vi "9045_sm.vi"() -> ()   [LabVIEW 2020]
uses:
  controls/sm_cluster.ctl
  controls/enum.ctl
  lib/labviewRT-EPICS/sm bool read and increment.vi
  lib/labviewRT-EPICS/sm bool write and increment.vi
  lib/labviewRT-EPICS/sm bool array write and increment.vi
  lib/labviewRT-EPICS/sm double read and increment.vi
  lib/labviewRT-EPICS/sm double write and increment.vi
  lib/labviewRT-EPICS/sm double array write and increment.vi
  lib/labviewRT-EPICS/sm i8 read and increment.vi
  lib/labviewRT-EPICS/sm i8 write and increment.vi
  lib/labviewRT-EPICS/sm i8 write array and increment.vi
  lib/labviewRT-EPICS/sm i16 read and increment.vi
  lib/labviewRT-EPICS/sm i16 write and increment.vi
  lib/labviewRT-EPICS/sm i16 write array and increment.vi
  lib/labviewRT-EPICS/sm i32 read and increment.vi
  lib/labviewRT-EPICS/sm i32 write and increment.vi
  lib/labviewRT-EPICS/sm i32 write array and increment.vi
  lib/labviewRT-EPICS/sm i64 read and increment.vi
  lib/labviewRT-EPICS/sm i64 write and increment.vi
  lib/labviewRT-EPICS/sm i64 write array and increment.vi
  lib/labviewRT-EPICS/sm single read and increment.vi
  lib/labviewRT-EPICS/sm single write and increment.vi
  lib/labviewRT-EPICS/sm single array write and increment.vi
  lib/labviewRT-EPICS/sm u8 read and increment.vi
  lib/labviewRT-EPICS/sm u8 write and increment.vi
  lib/labviewRT-EPICS/sm u8 write array and increment.vi
  lib/labviewRT-EPICS/sm u16 read and increment.vi
  lib/labviewRT-EPICS/sm u16 write and increment.vi
  lib/labviewRT-EPICS/sm u16 write array and increment.vi
  lib/labviewRT-EPICS/sm u32 read and increment.vi
  lib/labviewRT-EPICS/sm u32 write and increment.vi
  lib/labviewRT-EPICS/sm u32 write array and increment.vi
  lib/labviewRT-EPICS/sm u64 read and increment.vi
  lib/labviewRT-EPICS/sm u64 write and increment.vi
  lib/labviewRT-EPICS/sm u64 write array and increment.vi
  lib/labviewRT-EPICS/sm mbbi write and increment.vi
  lib/labviewRT-EPICS/sm mbbo read and increment.vi
  lib/labviewRT-EPICS/linuxSharedMemory.lvlib
panel:
  in  "d40":T1
  out "d41":T1
  out "d37":u64
  in  "d38":u64
  in  "d39":u64[](array[numeric])
  out "d34":u32
  in  "d35":u32
  in  "d36":u32[](array[numeric])
  out "d30":u16
  in  "d31":u16
  in  "d32":u16[](array[numeric])
  out "d26":u8
  in  "d27":u8
  in  "d28":u8[](array[numeric])
  out "d22":sgl format="%.2f"
  in  "d23":sgl
  in  "d24":sgl[](array[numeric])
  out "d18":i64
  in  "d19":i64
  in  "d20":i64[](array[numeric])
  out "d14":i32
  in  "d15":i32
  in  "d16":i32[](array[numeric])
  out "d10":i16
  in  "d11":i16
  in  "d12":i16[](array[numeric])
  out "d6":i8
  in  "d7":i8
  in  "d8":i8[](array[numeric])
  in  "d4":dbl[](array[numeric])
  in  "d3":dbl
  out "d2":dbl
  in  "boolArrayWrite":bool[](array[boolean])
  in  "value in":bool
  out "Shared memory cluster":T2
  out "Bool out":bool
  in  "stop":bool
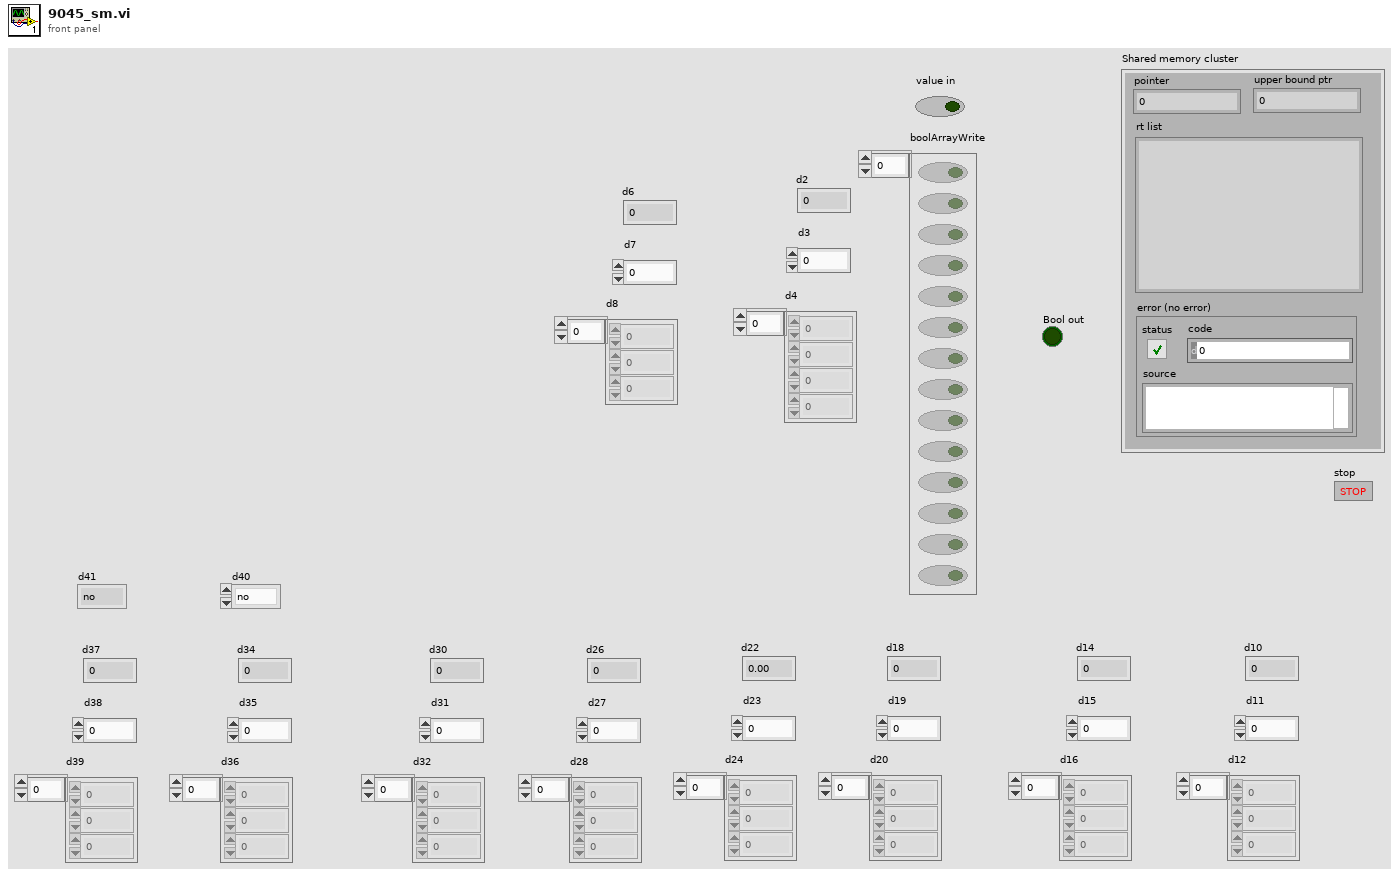
[diagram p1: front panel]
types:
  T1 = typedef "enum.ctl" = enum16{"no", "yes", "dont know"}
  T2 = typedef "linuxSharedMemory.lvlib/sm_cluster.ctl" = cluster{"rt list":string, "error (no error)":errorcluster, "pointer":u64, "upper bound ptr":u64}
  T3 = typedef "Linux RT IPC.Shared Memory.lvlib/reference.ctl" = refnum<data-value>
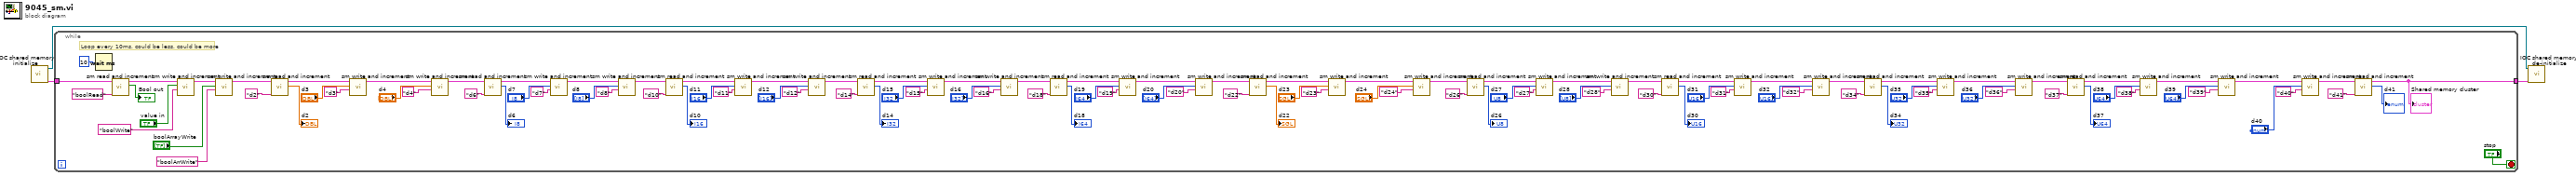
[diagram p0: block diagram]
diagram:
  n1 = call "IOC shared memory initialize.vi"() -> ("Shared memory cluster"=w2:T2, "shared memory class"=w3:T3)  [unwired: 10 in]
  n2 = while {
    tunnel: w2 -> [w21]
    tunnel: [w6] -> w1
    stop <- "stop" stop-if-true
    # "Loop every 10ms, could be less, could be more"
    n3 = Wait (ms)(milliseconds to wait=10) -> ()  [unwired: 1 out]
    n4 = call-poly "sm read and increment.vi"("Identifier"="boolRead", "Shared memory cluster input"=w21) -> ("Bool out"=→"Bool out":bool, "Shared memory cluster output"=w107:T2)  [unwired: 8 in]
    n5 = call-poly "sm write and increment.vi"("Identifier"="boolWrite", "value in"="value in", "Shared memory cluster input"=w107) -> ("Shared memory cluster output"=w104:T2)  [unwired: 8 in]
    n6 = call-poly "sm write and increment.vi"("Identifier"="boolArrWrite", "value in"="boolArrayWrite", "Shared memory cluster"=w104) -> ("Shared memory cluster output"=w20:T2)  [unwired: 8 in]
    n7 = call-poly "sm read and increment.vi"("Identifier"="d2", "Shared memory cluster input"=w20) -> ("Value out"=→"d2":dbl, "Shared memory cluster output"=w100:T2)  [unwired: 8 in]
    n8 = call-poly "sm write and increment.vi"("Identifier"="d3", "value in"="d3", "Shared memory cluster input"=w100) -> ("Shared memory cluster output"=w101:T2)  [unwired: 8 in]
    n9 = call-poly "sm write and increment.vi"("Identifier"="d4", "value in"="d4", "Shared memory cluster"=w101) -> ("Shared memory cluster output"=w19:T2)  [unwired: 8 in]
    n10 = call-poly "sm read and increment.vi"("Identifier"="d6", "Shared memory cluster input"=w19) -> ("Value out"=→"d6":i8, "Shared memory cluster output"=w92:T2)  [unwired: 8 in]
    n11 = call-poly "sm write and increment.vi"("Identifier"="d7", "value in"="d7", "Shared memory cluster input"=w92) -> ("Shared memory cluster output"=w93:T2)  [unwired: 8 in]
    n12 = call-poly "sm write and increment.vi"("Identifier"="d8", "value in"="d8", "Shared memory cluster"=w93) -> ("Shared memory cluster output"=w18:T2)  [unwired: 8 in]
    n13 = call-poly "sm read and increment.vi"("Identifier"="d10", "Shared memory cluster input"=w18) -> ("Value out"=→"d10":i16, "Shared memory cluster output"=w84:T2)  [unwired: 8 in]
    n14 = call-poly "sm write and increment.vi"("Identifier"="d11", "value in"="d11", "Shared memory cluster input"=w84) -> ("Shared memory cluster output"=w85:T2)  [unwired: 8 in]
    n15 = call-poly "sm write and increment.vi"("Identifier"="d12", "value in"="d12", "Shared memory cluster"=w85) -> ("Shared memory cluster output"=w17:T2)  [unwired: 8 in]
    n16 = call-poly "sm read and increment.vi"("Identifier"="d14", "Shared memory cluster input"=w17) -> ("Value out"=→"d14":i32, "Shared memory cluster output"=w76:T2)  [unwired: 8 in]
    n17 = call-poly "sm write and increment.vi"("Identifier"="d15", "value in"="d15", "Shared memory cluster input"=w76) -> ("Shared memory cluster output"=w77:T2)  [unwired: 8 in]
    n18 = call-poly "sm write and increment.vi"("Identifier"="d16", "value in"="d16", "Shared memory cluster"=w77) -> ("Shared memory cluster output"=w16:T2)  [unwired: 8 in]
    n19 = call-poly "sm read and increment.vi"("Identifier"="d18", "Shared memory cluster input"=w16) -> ("Value out"=→"d18":i64, "Shared memory cluster output"=w68:T2)  [unwired: 8 in]
    n20 = call-poly "sm write and increment.vi"("Identifier"="d19", "value in"="d19", "Shared memory cluster input"=w68) -> ("Shared memory cluster output"=w69:T2)  [unwired: 8 in]
    n21 = call-poly "sm write and increment.vi"("Identifier"="d20", "value in"="d20", "Shared memory cluster"=w69) -> ("Shared memory cluster output"=w15:T2)  [unwired: 8 in]
    n22 = call-poly "sm read and increment.vi"("Identifier"="d22", "Shared memory cluster input"=w15) -> ("Value out"=→"d22":sgl, "Shared memory cluster output"=w60:T2)  [unwired: 8 in]
    n23 = call-poly "sm write and increment.vi"("Identifier"="d23", "value in"="d23", "Shared memory cluster input"=w60) -> ("Shared memory cluster output"=w61:T2)  [unwired: 8 in]
    n24 = call-poly "sm write and increment.vi"("Identifier"="d24", "value in"="d24", "Shared memory cluster"=w61) -> ("Shared memory cluster output"=w14:T2)  [unwired: 8 in]
    n25 = call-poly "sm read and increment.vi"("Identifier"="d26", "Shared memory cluster input"=w14) -> ("Value out"=→"d26":u8, "Shared memory cluster output"=w52:T2)  [unwired: 8 in]
    n26 = call-poly "sm write and increment.vi"("Identifier"="d27", "value in"="d27", "Shared memory cluster input"=w52) -> ("Shared memory cluster output"=w53:T2)  [unwired: 8 in]
    n27 = call-poly "sm write and increment.vi"("Identifier"="d28", "value in"="d28", "Shared memory cluster"=w53) -> ("Shared memory cluster output"=w13:T2)  [unwired: 8 in]
    n28 = call-poly "sm read and increment.vi"("Identifier"="d30", "Shared memory cluster input"=w13) -> ("Value out"=→"d30":u16, "Shared memory cluster output"=w44:T2)  [unwired: 8 in]
    n29 = call-poly "sm write and increment.vi"("Identifier"="d31", "value in"="d31", "Shared memory cluster input"=w44) -> ("Shared memory cluster output"=w45:T2)  [unwired: 8 in]
    n30 = call-poly "sm write and increment.vi"("Identifier"="d32", "value in"="d32", "Shared memory cluster"=w45) -> ("Shared memory cluster output"=w11:T2)  [unwired: 8 in]
    n31 = call-poly "sm read and increment.vi"("Identifier"="d34", "Shared memory cluster input"=w11) -> ("Value out"=→"d34":u32, "Shared memory cluster output"=w36:T2)  [unwired: 8 in]
    n32 = call-poly "sm write and increment.vi"("Identifier"="d35", "value in"="d35", "Shared memory cluster input"=w36) -> ("Shared memory cluster output"=w37:T2)  [unwired: 8 in]
    n33 = call-poly "sm write and increment.vi"("Identifier"="d36", "value in"="d36", "Shared memory cluster"=w37) -> ("Shared memory cluster output"=w12:T2)  [unwired: 8 in]
    n34 = call-poly "sm read and increment.vi"("Identifier"="d37", "Shared memory cluster input"=w12) -> ("Value out"=→"d37":u64, "Shared memory cluster output"=w28:T2)  [unwired: 8 in]
    n35 = call-poly "sm write and increment.vi"("Identifier"="d38", "value in"="d38", "Shared memory cluster input"=w28) -> ("Shared memory cluster output"=w29:T2)  [unwired: 8 in]
    n36 = call-poly "sm write and increment.vi"("Identifier"="d39", "value in"="d39", "Shared memory cluster"=w29) -> ("Shared memory cluster output"=w10:T2)  [unwired: 8 in]
    n37 = call-poly "sm write and increment.vi"("Identifier"="d40", "value in"="d40", "Shared memory cluster input"=w10) -> ("Shared memory cluster output"=w7:T2)  [unwired: 8 in]
    n38 = call-poly "sm read and increment.vi"("Identifier"="d41", "Shared memory cluster input"=w7) -> ("Value out"=→"d41":u16, "Shared memory cluster output"=w6:T2)  [unwired: 8 in]
    "Shared memory cluster" <- w6
  }
  n39 = call "IOC shared memory de-initialize.vi"("shared memory in"=w3, "Shared memory cluster"=w1) -> ()  [unwired: 9 in]
